vi "Set Configuration.vi"(8 "error in (no error)":errorcluster, 11 "Analog PWM Input in":refnum<class "Analog PWM Input.lvclass">) -> (0 "error out":errorcluster, 3 "Analog PWM Input out":refnum<class "Analog PWM Input.lvclass">)   [LabVIEW 2015, in "Analog PWM Input.lvclass"]
uses:
  Analog PWM Input.lvclass
  IO Class/Type.ctl
  FPGA Addon Input/FPGA Addon Input.lvclass
  IO Class/IO Class.lvclass
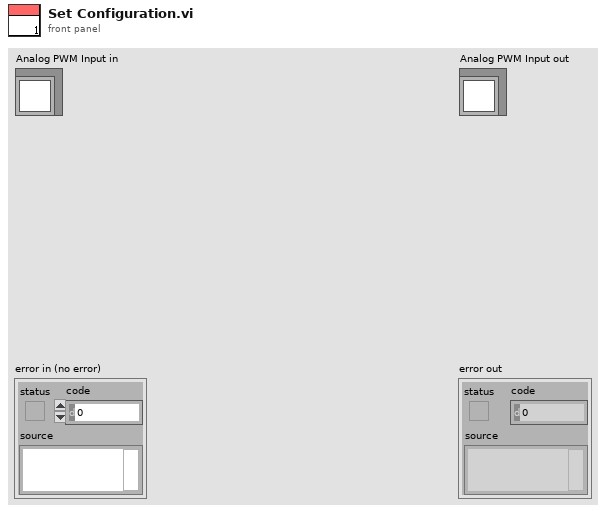
[diagram p1: front panel]
types:
  T1 = typedef "IO Class.lvclass/Type.ctl" = cluster{"Type":string}
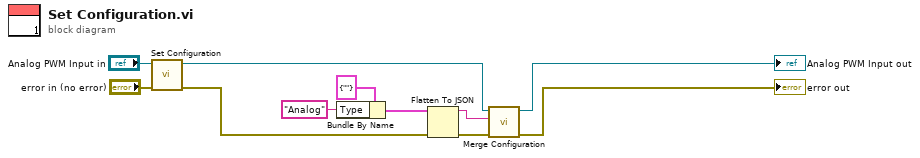
[diagram p0: block diagram]
diagram:
  n1 = call-parent "Set Configuration.vi"("error in (no error)"="error in (no error)", "FPGA Addon Input in"="Analog PWM Input in") -> ("error out"=w2:errorcluster, "FPGA Addon Input out"=w1:refnum<class "Analog PWM Input.lvclass">)  [unwired: 8 in]
  n2 = Bundle By Name(cluster=T1 {"Type"=""} ("Type"), "Type"="Analog") -> (w8:T1)
  n3 = Flatten To JSON(anything=w8, error in (no error)=w2) -> (JSON string=w6:string, 11:w5:errorcluster)  [unwired: 1 in]
  n4 = call "Merge Configuration.vi"("error in (no error)"=w5, "Additional Configuration"=w6, "IO Class in"=w1) -> ("error out"=→"error out":errorcluster, "IO Class out"=→"Analog PWM Input out":refnum<class "Analog PWM Input.lvclass">)  [unwired: 7 in]
